vi "log analysis_gps.vi"() -> ()   [LabVIEW 2018] (continued)
log_raw\tgps_raw\t\tsystem status\tnormal 2 28.300000 0 0\trobot status\t14.669720\t18.434430\t9.580100\t-0.442703\t-1.332140\t56.640484\t0.481000\t-0.012000\n\t\n15:06:21.6\tlog_raw\tgps_raw\t\tsystem status\tnormal 2 28.300000 0 0\trobot status\t14.797529\t18.634109\t9.573000\t-0.410192\t-1.362528\t56.475857\t0.491000\t-0.012000\n\t\n15:06:22.1\tlog_raw\tgps_raw\t\tsystem status\tnormal 2 28.300000 0 0\trobot status\t14.927663\t18.831915\t9.567300\t-0.251703\t-1.268455\t56.075924\t0.492000\t-0.025000\n\t\n15:06:22.6\tlog_raw\tgps_raw\t\tsystem status\tnormal 2 28.200000 0 0\trobot status\t15.059315\t19.031378\t9.560500\t-0.198157\t-1.501771\t56.406784\t0.493000\t-0.027000\n\t\n15:06:23.1\tlog_raw\tgps_raw\t\tsystem status\tnormal 2 28.300000 0 0\trobot status\t15.196538\t19.238415\t9.553100\t-0.161311\t-1.683922\t55.984398\t0.499000\t-0.017000\n\t\n15:06:23.6\tlog_raw\tgps_raw\t\tsystem status\tnormal 2 28.300000 0 0\trobot status\t15.328121\t19.432271\t9.546000\t-0.255888\t-1.624208\t55.884857\t0.485000\t-0.045000\n\t\n15:06:24.1\tlog_raw\tgps_raw\t\tsystem status\tnormal 2 28.300000 0 0\trobot status\t15.462626\t19.627022\t9.539100\t-0.210675\t-1.326281\t55.617352\t0.516000\t-0.008000\n\t\n15:06:24.6\tlog_raw\tgps_raw\t\tsystem status\tnormal 2 28.300000 0 0\trobot status\t15.603892\t19.828177\t9.530800\t-0.413985\t-1.434365\t55.397999\t0.465000\t-0.076000\n\t\n15:06:25.1\tlog_raw\tgps_raw\t\tsystem status\tnormal 2 28.200000 0 0\trobot status\t15.741500\t20.019302\t9.525900\t-0.572236\t-1.445230\t54.718037\t0.467000\t-0.089000\n\t\n15:06:25.6\tlog_raw\tgps_raw\t\tsystem status\tnormal 2 28.200000 0 0\trobot status\t15.882218\t20.207334\t9.519900\t-0.498192\t-1.514932\t54.414841\t0.447000\t-0.134000\n\t\n15:06:26.1\tlog_raw\tgps_raw\t\tsystem status\tnormal 2 28.200000 0 0\trobot status\t16.023898\t20.392153\t9.513000\t-0.472443\t-1.210385\t53.436024\t0.532000\t0.043000\n\t\n15:06:26.7\tlog_raw\tgps_raw\t\tsystem status\tnormal 2 28.200000 0 0\trobot status\t16.171592\t20.578219\t9.506200\t-0.708328\t-1.308049\t52.570660\t0.594000\t0.124000\n\t\n15:06:27.1\tlog_raw\tgps_raw\t\tsystem status\tnormal 2 28.200000 0 0\trobot status\t16.321970\t20.758672\t9.499000\t-0.603389\t-1.161147\t50.202438\t0.716000\t0.307000\n\t\n15:06:27.7\tlog_raw\tgps_raw\t\tsystem status\tnormal 2 28.200000 0 0\trobot status\t16.472637\t20.937047\t9.494000\t-0.823952\t-1.192068\t49.516270\t0.549000\t0.052000\n\t\n15:06:28.2\tlog_raw\tgps_raw\t\tsystem status\tnormal 2 28.300000 0 0\trobot status\t16.626209\t21.110847\t9.487200\t-0.618338\t-1.040485\t49.357948\t0.445000\t-0.079000\n\t\n15:06:28.7\tlog_raw\tgps_raw\t\tsystem status\tnormal 2 28.300000 0 0\trobot status\t16.782273\t21.286651\t9.481200\t-0.644616\t-1.219018\t49.316982\t0.467000\t-0.020000\n\t\n15:06:29.2\tlog_raw\tgps_raw\t\tsystem status\tnormal 2 28.300000 0 0\trobot status\t16.937583\t21.455267\t9.475200\t-0.611529\t-1.254126\t50.028496\t0.494000\t0.009000\n\t\n15:06:29.7\tlog_raw\tgps_raw\t\tsystem status\tnormal 2 28.300000 0 0\trobot status\t17.093303\t21.621011\t9.474500\t-0.765682\t-0.913837\t48.514305\t0.492000\t0.019000\n\t\n15:06:30.2\tlog_raw\tgps_raw\t\tsystem status\tnormal 2 28.200000 0 0\trobot status\t17.247377\t21.778171\t9.473400\t-0.418232\t-0.521781\t48.645527\t0.503000\t0.018000\n\t\n15:06:30.7\tlog_raw\tgps_raw\t\tsystem status\tnormal 2 28.300000 0 0\trobot status\t17.414327\t21.954053\t9.468700\t-0.366987\t-0.668392\t48.759113\t0.491000\t0.027000\n\t\n15:06:31.2\tlog_raw\tgps_raw\t\tsystem status\tnormal 2 28.300000 0 0\trobot status\t17.576209\t22.121930\t9.465900\t-0.344665\t-0.985004\t48.117779\t0.514000\t0.007000\n\t\n15:06:31.7\tlog_raw\tgps_raw\t\tsystem status\tnormal 2 28.200000 0 0\trobot status\t17.741651\t22.297663\t9.462100\t-0.296414\t-1.204172\t48.951267\t0.600000\t-0.140000\n\t\n15:06:32.2\tlog_raw\tgps_raw\t\tsystem status\tnormal 2 28.200000 0 0\trobot status\t17.899739\t22.464471\t9.457900\t-0.150727\t-1.166923\t49.356468\t0.469000\t0.059000\n\t\n15:06:32.7\tlog_raw\tgps_raw\t\tsystem status\tnormal 2 28.100000 0 0\trobot status\t18.056766\t22.634728\t9.453400\t-0.116821\t-1.019282\t49.798592\t0.340000\t0.260000\n\t\n15:06:33.2\tlog_raw\tgps_raw\t\tsystem status\tnormal 2 28.100000 0 0\trobot status\t18.210251\t22.807417\t9.449800\t-0.101973\t-1.178444\t51.238773\t0.429000\t0.127000\n\t\n15:06:33.7\tlog_raw\tgps_raw\t\tsystem status\tnormal 2 28.000000 0 0\trobot status\t18.356919\t22.986067\t9.447300\t-0.277614\t-0.965312\t52.540962\t0.440000\t0.150000\n\t\n15:06:34.2\tlog_raw\tgps_raw\t\tsystem status\tnormal 2 28.000000 0 0\trobot status\t18.501103\t23.165006\t9.443600\t-0.171265\t-0.728076\t53.288834\t0.541000\t-0.049000\n\t\n15:06:34.7\tlog_raw\tgps_raw\t\tsystem status\tnormal 2 28.000000 0 0\trobot status\t18.643616\t23.349578\t9.441700\t0.001085\t-0.423099\t53.132992\t0.514000\t0.022000\n\t\n15:06:35.2\tlog_raw\tgps_raw\t#INSPVAXA,USB3,0,46.0,FINESTEERING,2107,281213.200,02000000,471d,15824;INS_ALIGNMENT_COMPLETE,INS_RTKFIXED,37.37034248828,126.72104733937,9.4372,22.3000,0.3538,0.2828,-0.0066,-0.047417832,-0.921096581,33.030780254,0.4120,0.2924,0.5519,0.1133,0.0939,0.0858,0.2818,0.2696,4.9671,0f000001,0*5574abbc\n\tsystem status\tnormal 2 28.000000 0 0\trobot status\t18.799365\t23.561095\t9.437200\t-0.047418\t-0.921097\t53.638321\t0.558000\t-0.089000\n\t\n15:06:35.7\tlog_raw\tgps_raw\t\tsystem status\tnormal 2 28.000000 0 0\trobot status\t18.923249\t23.736439\t9.433200\t-0.135144\t-1.055623\t54.359356\t0.640000\t-0.194000\n\t\n15:06:36.2\tlog_raw\tgps_raw\t\tsystem status\tnormal 2 28.100000 0 0\trobot status\t19.058113\t23.933319\t9.428500\t-0.205469\t-1.114172\t54.854160\t0.442000\t0.079000\n\t\n15:06:36.7\tlog_raw\tgps_raw\t\tsystem status\tnormal 2 28.100000 0 0\trobot status\t19.188419\t24.132723\t9.424800\t-0.121815\t-0.847459\t55.364796\t0.450000\t0.092000\n\t\n15:06:37.2\tlog_raw\tgps_raw\t#INSPVAXA,USB3,0,45.5,FINESTEERING,2107,281215.200,02000000,471d,15824;INS_ALIGNMENT_COMPLETE,INS_RTKFIXED,37.37034967081,126.72105335114,9.4206,22.3000,0.3913,0.2859,-0.0158,-0.209950038,-1.067150096,30.856231444,0.4131,0.2932,0.5613,0.1129,0.0941,0.0863,0.2814,0.2689,4.9698,0f000001,0*15a1dcfe\n\tsystem status\tnormal 2 28.200000 0 0\trobot status\t19.331878\t24.358244\t9.420600\t-0.209950\t-1.067150\t56.490650\t0.418000\t0.124000\n\t\n15:06:37.7\tlog_raw\tgps_raw\t\tsystem status\tnormal 2 28.200000 0 0\trobot status\t19.448752\t24.543859\t9.415800\t-0.435181\t-1.200392\t56.363674\t0.656000\t-0.251000\n\t\n15:06:38.2\tlog_raw\tgps_raw\t\tsystem status\tnormal 2 28.200000 0 0\trobot status\t19.578892\t24.747485\t9.410400\t-0.394118\t-1.104838\t56.147427\t0.483000\t0.009000\n\t\n15:06:38.7\tlog_raw\tgps_raw\t\tsystem status\tnormal 2 28.200000 0 0\trobot status\t19.708910\t24.951700\t9.408000\t-0.473816\t-0.971366\t56.946445\t0.453000\t0.039000\n\t\n15:06:39.2\tlog_raw\tgps_raw\t\tsystem status\tnormal 2 28.200000 0 0\trobot status\t19.839004\t25.154821\t9.405200\t-0.424478\t-1.089783\t55.912186\t0.480000\t0.003000\n\t\n15:06:39.7\tlog_raw\tgps_raw\t#INSPVAXA,USB3,0,47.5,FINESTEERING,2107,281217.700,02000000,471d,15824;INS_ALIGNMENT_COMPLETE,INS_RTKFIXED,37.37035891275,126.72106070272,9.4027,22.3000,0.3907,0.2751,-0.0370,-0.475151732,-0.956253222,31.086527744,0.4118,0.2907,0.5637,0.1115,0.0927,0.0836,0.2812,0.2687,4.9728,0f000001,0*c5b8ff8b\n\tsystem status\tnormal 2 28.300000 0 0\trobot status\t19.983069\t25.383955\t9.402700\t-0.475152\t-0.956253\t55.553867\t0.493000\t-0.013000\n\t\n15:06:40.2\tlog_raw\tgps_raw\t\tsystem status\tnormal 2 28.300000 0 0\trobot status\t20.097932\t25.563951\t9.402700\t-0.538281\t-0.688897\t56.219219\t0.499000\t-0.015000\n\t\n15:06:40.7\tlog_raw\tgps_raw\t#INSPVAXA,USB3,0,41.5,FINESTEERING,2107,281218.700,02000000,471d,15824;INS_ALIGNMENT_COMPLETE,INS_RTKFIXED,37.37036254864,126.72106366487,9.4005,22.3000,0.3951,0.2706,-0.0129,-0.403197852,-0.697835271,31.463679771,0.4109,0.2895,0.5628,0.1119,0.0933,0.0832,0.2811,0.2686,4.9743,0f000001,0*95cb54ca\n\tsystem status\tnormal 2 28.200000 0 0\trobot status\t20.245451\t25.787482\t9.400500\t-0.403198\t-0.697835\t55.319050\t0.493000\t-0.022000\n\t\n15:06:41.2\tlog_raw\tgps_raw\t\tsystem status\tnormal 2 28.200000 0 0\trobot status\t20.362973\t25.969116\t9.399600\t-0.606996\t-0.535913\t56.163181\t0.494000\t-0.027000\n\t\n15:06:41.7\tlog_raw\tgps_raw\t\tsystem status\tnormal 2 28.300000 0 0\trobot status\t20.493689\t26.170169\t9.401200\t-0.861722\t-0.670275\t55.873943\t0.502000\t-0.039000\n\t\n15:06:42.2\tlog_raw\tgps_raw\t\tsystem status\tnormal 2 28.300000 0 0\trobot status\t20.632432\t26.380765\t9.400800\t-0.844302\t-0.845400\t54.259411\t0.490000\t-0.026000\n\t\n15:06:42.7\tlog_raw\tgps_raw\t#INSPVAXA,USB3,0,45.0,FINESTEERING,2107,281220.700,02000000,471d,15824;INS_ALIGNMENT_COMPLETE,INS_RTKFIXED,37.37036990061,126.72106971349,9.4025,22.3000,0.4109,0.2911,0.0071,-0.800702945,-0.878644990,32.737645043,0.4094,0.2870,0.5571,0.1117,0.0929,0.0807,0.2810,0.2681,4.9772,0f000001,0*67c969e8\n\tsystem status\tnormal 2 28.200000 0 0\trobot status\t20.781228\t26.603436\t9.402500\t-0.800703\t-0.878645\t54.810455\t0.511000\t-0.023000\n\t\n15:06:43.2\tlog_raw\tgps_raw\t#INSPVAXA,USB3,0,42.5,FINESTEERING,2107,281221.200,02000000,471d,15824;INS_ALIGNMENT_COMPLETE,INS_RTKFIXED,37.37037172466,126.72107126440,9.4031,22.3000,0.4112,0.2890,-0.0190,-0.732165245,-0.750314239,33.130718379,0.4093,0.2853,0.5533,0.1117,0.0926,0.0797,0.2808,0.2678,4.9785,0f000001,0*69bb78c8\n\tsystem status\tnormal 2 28.200000 0 0\trobot status\t20.918605\t26.805878\t9.403100\t-0.732165\t-0.750314\t53.298634\t0.499000\t-0.017000\n\t\n15:06:43.7\tlog_raw\tgps_raw\t\tsystem status\tnormal 2 28.200000 0 0\trobot status\t21.046031\t26.987368\t9.403400\t-0.631340\t-0.757970\t54.422825\t0.498000\t-0.011000\n\t\n15:06:44.2\tlog_raw\tgps_raw\t\tsystem status\tnormal 2 28.200000 0 0\trobot status\t21.184536\t27.183020\t9.401900\t-0.652815\t-0.900259\t53.609329\t0.446000\t-0.086000\n\t\n15:06:44.7\tlog_raw\tgps_raw\t\tsystem status\tnormal 2 28.300000 0 0\trobot status\t21.325364\t27.376921\t9.402200\t-0.694030\t-0.892817\t53.428085\t0.543000\t0.053000\n\t\n15:06:45.2\tlog_raw\tgps_raw\t\tsystem status\tnormal 2 28.200000 0 0\trobot status\t21.469638\t27.569712\t9.402700\t-0.559469\t-0.735313\t52.854458\t0.654000\t0.219000\n\t\n15:06:45.7\tlog_raw\tgps_raw\t\tsystem status\tnormal 2 28.200000 0 0\trobot status\t21.616373\t27.759644\t9.402600\t-0.651466\t-0.781679\t51.706299\t0.653000\t0.201000\n\t\n15:06:46.2\tlog_raw\tgps_raw\t\tsystem status\tnormal 2 28.200000 0 0\trobot status\t21.764966\t27.945708\t9.403800\t-0.588520\t-0.809740\t51.243496\t0.562000\t0.068000\n\t\n15:06:46.7\tlog_raw\tgps_raw\t#INSPVAXA,USB3,0,47.0,FINESTEERING,2107,281224.700,02000000,471d,15824;INS_ALIGNMENT_COMPLETE,INS_RTKFIXED,37.37038378890,126.72108266803,9.4041,22.3000,0.3641,0.2986,-0.0101,-0.663611718,-0.597748671,37.087466475,0.4089,0.2830,0.5420,0.1122,0.0925,0.0797,0.2801,0.2667,4.9821,0f000001,0*d2353e58\n\tsystem status\tnormal 2 28.200000 0 0\trobot status\t21.928720\t28.144820\t9.404100\t-0.663612\t-0.597749\t50.318630\t0.431000\t-0.109000\n\t\n15:06:47.2\tlog_raw\tgps_raw\t\tsystem status\tnormal 2 28.200000 0 0\trobot status\t22.067987\t28.309838\t9.404300\t-0.492724\t-0.435729\t50.359184\t0.490000\t-0.020000\n\t\n15:06:47.7\tlog_raw\tgps_raw\t#INSPVAXA,USB3,0,49.0,FINESTEERING,2107,281225.700,02008000,471d,15824;INS_ALIGNMENT_COMPLETE,INS_RTKFIXED,37.37038703252,126.72108609198,9.4018,22.3000,0.3794,0.3187,-0.0066,-0.623620259,-0.927536897,37.861250178,0.4087,0.2831,0.5398,0.1124,0.0928,0.0802,0.2799,0.2664,4.9834,0f000001,0*fbb2d3ef\n\tsystem status\tnormal 2 28.200000 0 0\trobot status\t22.232008\t28.504811\t9.401800\t-0.623620\t-0.927537\t49.387749\t0.499000\t-0.009000\n\t\n15:06:48.2\tlog_raw\tgps_raw\t\tsystem status\tnormal 2 28.200000 0 0\trobot status\t22.365284\t28.660268\t9.401600\t-0.754168\t-1.309650\t49.058773\t0.479000\t0.009000\n\t\n15:06:48.7\tlog_raw\tgps_raw\t#INSPVAXA,USB3,0,46.0,FINESTEERING,2107,281226.700,02008000,471d,15824;INS_ALIGNMENT_COMPLETE,INS_RTKFIXED,37.37039019698,126.72108954824,9.4032,22.3000,0.3584,0.3195,-0.0134,-0.717043811,-1.235643045,38.442839555,0.4087,0.2833,0.5380,0.1119,0.0921,0.0796,0.2798,0.2663,4.9847,0f000001,0*b92bfc16\n\tsystem status\tnormal 2 28.300000 0 0\trobot status\t22.538157\t28.856016\t9.403200\t-0.717044\t-1.235643\t49.151516\t0.493000\t0.009000\n\t\n15:06:49.2\tlog_raw\tgps_raw\t\tsystem status\tnormal 2 28.300000 0 0\trobot status\t22.678868\t29.011378\t9.400800\t-0.623594\t-1.018401\t49.199638\t0.496000\t0.016000\n\t\n15:06:49.7\tlog_raw\tgps_raw\t#INSPVAXA,USB3,0,43.5,FINESTEERING,2107,281227.700,02008000,471d,15824;INS_ALIGNMENT_COMPLETE,INS_RTKFIXED,37.37039325687,126.72109307012,9.3982,22.3000,0.3516,0.3055,0.0005,-0.625802804,-1.271897010,38.869801853,0.4083,0.2827,0.5361,0.1122,0.0924,0.0800,0.2797,0.2662,4.9860,0f000001,0*e8201bda\n\tsystem status\tnormal 2 28.300000 0 0\trobot status\t22.850120\t29.195616\t9.398200\t-0.625803\t-1.271897\t48.625996\t0.493000\t0.011000\n\t\n15:06:50.2\tlog_raw\tgps_raw\t#INSPVAXA,USB3,0,44.5,FINESTEERING,2107,281228.200,02008000,471d,15824;INS_ALIGNMENT_COMPLETE,INS_RTKFIXED,37.37039486129,126.72109491850,9.3967,22.3000,0.3668,0.3505,-0.0187,-0.688902140,-1.335982228,38.955777552,0.4076,0.2823,0.5343,0.1119,0.0921,0.0794,0.2796,0.2660,4.9872,0f000001,0*8630753c\n\tsystem status\tnormal 2 28.300000 0 0\trobot status\t23.013846\t29.373682\t9.396700\t-0.688902\t-1.335982\t48.590324\t0.506000\t0.017000\n\t\n15:06:50.7\tlog_raw\tgps_raw\t\tsystem status\tnormal 2 28.200000 0 0\trobot status\t23.159327\t29.527717\t9.396200\t-0.419608\t-1.258090\t48.867809\t0.419000\t0.117000\n\t\n15:06:51.2\tlog_raw\tgps_raw\t#INSPVAXA,USB3,0,42.5,FINESTEERING,2107,281229.200,02008000,471d,15824;INS_ALIGNMENT_COMPLETE,INS_RTKFIXED,37.37039793167,126.72109852773,9.3953,22.3000,0.3279,0.2928,-0.0255,-0.253376052,-0.991820405,38.455195972,0.4075,0.2825,0.5342,0.1118,0.0921,0.0790,0.2795,0.2658,4.9885,0f000001,0*8eb4cf39\n\tsystem status\tnormal 2 28.200000 0 0\trobot status\t23.333546\t29.714446\t9.395300\t-0.253376\t-0.991820\t50.004395\t0.514000\t-0.011000\n\t\n15:06:51.7\tlog_raw\tgps_raw\t#INSPVAXA,USB3,0,42.5,FINESTEERING,2107,281229.700,02008000,471d,15824;INS_ALIGNMENT_COMPLETE,INS_RTKFIXED,37.37039951050,126.72110026434,9.3940,22.3000,0.3314,0.2910,-0.0037,-0.337455745,-0.999192864,37.610056402,0.4075,0.2825,0.5342,0.1118,0.0921,0.0790,0.2795,0.2658,4.9885,0f000001,0*825b5af1\n\tsystem status\tnormal 2 28.100000 0 0\trobot status\t23.487372\t29.889671\t9.394000\t-0.337456\t-0.999193\t51.128315\t0.533000\t-0.026000\n\t\n15:06:52.2\tlog_raw\tgps_raw\t\tsystem status\tnormal 2 28.100000 0 0\trobot status\t23.625713\t30.049641\t9.393400\t-0.271176\t-1.130819\t51.201752\t0.436000\t0.112000\n\t\n15:06:52.7\tlog_raw\tgps_raw\t#INSPVAXA,USB3,0,48.0,FINESTEERING,2107,281230.700,02000000,471d,15824;INS_ALIGNMENT_COMPLETE,INS_RTKFIXED,37.37040272369,126.72110367197,9.3887,22.3000,0.3216,0.2986,0.0135,-0.067201953,-1.333373394,35.463092015,0.4076,0.2834,0.5341,0.1119,0.0922,0.0790,0.2794,0.2655,4.9897,0f000001,0*735b730c\n\tsystem status\tnormal 2 28.000000 0 0\trobot status\t23.789214\t30.246285\t9.388700\t-0.067202\t-1.333373\t52.971828\t0.415000\t0.157000\n\t\n15:06:53.2\tlog_raw\tgps_raw\t#INSPVAXA,USB3,0,47.0,FINESTEERING,2107,281231.200,02000000,471d,15824;INS_ALIGNMENT_COMPLETE,INS_RTKFIXED,37.37040437272,126.72110529054,9.3853,22.3000,0.3713,0.2903,-0.0029,0.017258070,-1.218794572,34.494374429,0.4079,0.2828,0.5329,0.1115,0.0914,0.0786,0.2791,0.2650,4.9910,0f000001,0*8245b70f\n\tsystem status\tnormal 2 28.000000 0 0\trobot status\t23.932585\t30.429301\t9.385300\t0.017258\t-1.218795\t53.613220\t0.408000\t0.170000\n\t\n15:06:53.7\tlog_raw\tgps_raw\t\tsystem status\tnormal 2 28.100000 0 0\trobot status\t24.056260\t30.599212\t9.380600\t-0.026863\t-1.285130\t55.009392\t0.549000\t-0.026000\n\t\n15:06:54.2\tlog_raw\tgps_raw\t#INSPVAXA,USB3,0,48.0,FINESTEERING,2107,281232.200,02000000,471d,15824;INS_ALIGNMENT_COMPLETE,INS_RTKFIXED,37.37040781109,126.72110834724,9.3744,22.3000,0.3888,0.2640,-0.0077,-0.124217348,-1.394698716,32.685462252,0.4076,0.2824,0.5319,0.1108,0.0907,0.0781,0.2788,0.2646,4.9925,0f000001,0*3486c657\n\tsystem status\tnormal 2 28.000000 0 0\trobot status\t24.203342\t30.810907\t9.374400\t-0.124217\t-1.394699\t55.228851\t0.325000\t0.271000\n\t\n15:06:54.7\tlog_raw\tgps_raw\t#INSPVAXA,USB3,0,48.0,FINESTEERING,2107,281232.700,02000000,471d,15824;INS_ALIGNMENT_COMPLETE,INS_RTKFIXED,37.37040957768,126.72110983569,9.3683,22.3000,0.3693,0.2541,-0.0175,-0.035465033,-1.483738306,31.883679858,0.4076,0.2824,0.5319,0.1108,0.0907,0.0781,0.2788,0.2646,4.9925,0f000001,0*4cf861df\n\tsystem status\tnormal 2 28.100000 0 0\trobot status\t24.335187\t31.006971\t9.368300\t-0.035465\t-1.483738\t55.660633\t0.385000\t0.203000\n\t\n15:06:55.2\tlog_raw\tgps_raw\t#INSPVAXA,USB3,0,42.5,FINESTEERING,2107,281233.200,02000000,471d,15824;INS_ALIGNMENT_COMPLETE,INS_RTKFIXED,37.37041136091,126.72111130172,9.3607,22.3000,0.3896,0.2699,-0.0002,0.128694926,-1.559285557,31.391109709,0.4078,0.2816,0.5308,0.1112,0.0913,0.0791,0.2786,0.2642,4.9941,0f000001,0*46ab5c2a\n\tsystem status\tnormal 2 28.100000 0 0\trobot status\t24.465045\t31.204881\t9.360700\t0.128695\t-1.559286\t56.024055\t0.428000\t0.097000\n\t\n15:06:55.7\tlog_raw\tgps_raw\t#INSPVAXA,USB3,0,42.5,FINESTEERING,2107,281233.700,02000000,471d,15824;INS_ALIGNMENT_COMPLETE,INS_RTKFIXED,37.37041314780,126.72111272697,9.3553,22.3000,0.3924,0.2487,-0.0281,0.163758724,-1.359425913,31.096827482,0.4078,0.2816,0.5308,0.1112,0.0913,0.0791,0.2786,0.2642,4.9941,0f000001,0*d64e85f7\n\tsystem status\tnormal 2 28.100000 0 0\trobot status\t24.591291\t31.403198\t9.355300\t0.163759\t-1.359426\t56.679836\t0.391000\t0.162000\n\t\n15:06:56.2\tlog_raw\tgps_raw\t#INSPVAXA,USB3,0,47.0,FINESTEERING,2107,281234.200,02000000,471d,15824;INS_ALIGNMENT_COMPLETE,INS_RTKFIXED,37.37041499218,126.72111417057,9.3481,22.3000,0.4102,0.2507,-0.0208,-0.006261741,-1.350650653,30.806533983,0.4074,0.2813,0.5302,0.1115,0.0918,0.0799,0.2784,0.2639,4.9958,0f000001,0*5fc48718\n\tsystem status\tnormal 2 28.200000 0 0\trobot status\t24.719163\t31.607896\t9.348100\t-0.006262\t-1.350651\t55.675377\t0.414000\t0.126000\n\t\n15:06:56.7\tlog_raw\tgps_raw\t#INSPVAXA,USB3,0,47.0,FINESTEERING,2107,281234.700,02000000,471d,15824;INS_ALIGNMENT_COMPLETE,INS_RTKFIXED,37.37041679366,126.72111558413,9.3430,22.3000,0.3853,0.2462,-0.0143,0.055762675,-1.167743160,30.720625161,0.4074,0.2813,0.5302,0.1115,0.0918,0.0799,0.2784,0.2639,4.9958,0f000001,0*9a377d3f\n\tsystem status\tnormal 2 28.200000 0 0\trobot status\t24.844374\t31.807832\t9.343000\t0.055763\t-1.167743\t57.176826\t0.404000\t0.142000\n\t\n15:06:57.2\tlog_raw\tgps_raw\t#INSPVAXA,USB3,0,48.0,FINESTEERING,2107,281235.200,02000000,471d,15824;INS_ALIGNMENT_COMPLETE,INS_RTKFIXED,37.37041862614,126.72111704485,9.3377,22.3000,0.3985,0.2540,-0.0201,0.294289103,-1.099012992,30.736583565,0.4070,0.2811,0.5299,0.1117,0.0922,0.0805,0.2783,0.2638,4.9972,0f000001,0*a95814ac\n\tsystem status\tnormal 2 28.200000 0 0\trobot status\t24.973762\t32.011208\t9.337700\t0.294289\t-1.099013\t57.295681\t0.594000\t-0.146000\n\t\n15:06:57.7\tlog_raw\tgps_raw\t\tsystem status\tnormal 2 28.300000 0 0\trobot status\t25.089206\t32.194708\t9.334000\t0.121491\t-1.212612\t57.047039\t0.475000\t0.029000\n\t\n15:06:58.2\tlog_raw\tgps_raw\t#INSPVAXA,USB3,0,44.0,FINESTEERING,2107,281236.200,02000000,471d,15824;INS_ALIGNMENT_COMPLETE,INS_RTKFIXED,37.37042228816,126.72111996191,9.3297,22.3000,0.3967,0.2694,0.0011,0.104811084,-1.415486457,30.958501575,0.4068,0.2811,0.5298,0.1121,0.0927,0.0811,0.2782,0.2636,4.9988,0f000001,0*e69fee41\n\tsystem status\tnormal 2 28.200000 0 0\trobot status\t25.232150\t32.417635\t9.329700\t0.104811\t-1.415486\t57.066120\t0.489000\t-0.015000\n\t\n15:06:58.7\tlog_raw\tgps_raw\t#INSPVAXA,USB3,0,44.0,FINESTEERING,2107,281236.700,02000000,471d,15824;INS_ALIGNMENT_COMPLETE,INS_RTKFIXED,37.37042410585,126.72112143606,9.3271,22.3000,0.4148,0.2479,-0.0173,0.069526094,-1.244882003,31.226949687,0.4068,0.2811,0.5298,0.1121,0.0927,0.0811,0.2782,0.2636,4.9988,0f000001,0*974dad1a\n\tsystem status\tnormal 2 28.200000 0 0\trobot status\t25.362728\t32.619371\t9.327100\t0.069526\t-1.244882\t57.115856\t0.494000\t-0.018000\n\t\n15:06:59.2\tlog_raw\tgps_raw\t#INSPVAXA,USB3,0,45.5,FINESTEERING,2107,281237.200,02000000,471d,15824;INS_ALIGNMENT_COMPLETE,INS_RTKFIXED,37.37042595037,126.72112294514,9.3228,22.3000,0.4143,0.2621,-0.0195,0.018984845,-1.146574514,31.412832351,0.4068,0.2809,0.5300,0.1124,0.0929,0.0818,0.2782,0.2635,5.0001,0f000001,0*1b0b7511\n\tsystem status\tnormal 2 28.300000 0 0\trobot status\t25.496400\t32.824083\t9.322800\t0.018985\t-1.146575\t56.291309\t0.494000\t-0.025000\n\t\n15:06:59.7\tlog_raw\tgps_raw\t\tsystem status\tnormal 2 28.300000 0 0\trobot status\t25.616064\t33.008512\t9.318600\t-0.220666\t-1.168167\t55.641972\t0.494000\t-0.031000\n\t\n15:07:00.2\tlog_raw\tgps_raw\t#INSPVAXA,USB3,0,46.0,FINESTEERING,2107,281238.200,02000000,471d,15824;INS_ALIGNMENT_COMPLETE,INS_RTKFIXED,37.37042950556,126.72112589522,9.3162,22.3000,0.4227,0.2698,0.0109,-0.200950173,-1.225682197,31.991269010,0.4072,0.2814,0.5306,0.1126,0.0929,0.0821,0.2781,0.2633,5.0015,0f000001,0*0794d365\n\tsystem status\tnormal 2 28.200000 0 0\trobot status\t25.757713\t33.218654\t9.316200\t-0.200950\t-1.225682\t55.934803\t0.493000\t-0.033000\n\t\n15:07:00.7\tlog_raw\tgps_raw\t#INSPVAXA,USB3,0,46.0,FINESTEERING,2107,281238.700,02000000,471d,15824;INS_ALIGNMENT_COMPLETE,INS_RTKFIXED,37.37043136222,126.72112745012,9.3124,22.3000,0.3943,0.2610,-0.0034,-0.386075100,-1.055396973,32.303525418,0.4072,0.2814,0.5306,0.1126,0.0929,0.0821,0.2781,0.2633,5.0015,0f000001,0*b83f878f\n\tsystem status\tnormal 2 28.300000 0 0\trobot status\t25.895444\t33.424714\t9.312400\t-0.386075\t-1.055397\t55.359413\t0.488000\t-0.027000\n\t\n15:07:01.2\tlog_raw\tgps_raw\t#INSPVAXA,USB3,0,48.0,FINESTEERING,2107,281239.200,02000000,471d,15824;INS_ALIGNMENT_COMPLETE,INS_RTKFIXED,37.37043317421,126.72112899719,9.3082,22.3000,0.4229,0.2915,-0.0051,-0.601506293,-1.130264131,32.679510223,0.4077,0.2817,0.5313,0.1126,0.0927,0.0822,0.2780,0.2630,5.0030,0f000001,0*20b6ea60\n\tsystem status\tnormal 2 28.200000 0 0\trobot status\t26.032481\t33.625817\t9.308200\t-0.601506\t-1.130264\t54.440792\t0.518000\t0.007000\n\t\n15:07:01.7\tlog_raw\tgps_raw\t#INSPVAXA,USB3,0,48.0,FINESTEERING,2107,281239.700,02000000,471d,15824;INS_ALIGNMENT_COMPLETE,INS_RTKFIXED,37.37043494669,126.72113055654,9.3053,22.3000,0.3888,0.2751,0.0114,-0.527038366,-1.080230445,33.250438434,0.4077,0.2817,0.5313,0.1126,0.0927,0.0822,0.2780,0.2630,5.0030,0f000001,0*94791092\n\tsystem status\tnormal 2 28.200000 0 0\trobot status\t26.170605\t33.822534\t9.305300\t-0.527038\t-1.080230\t54.062698\t0.518000\t0.028000\n\t\n15:07:02.2\tlog_raw\tgps_raw\t\tsystem status\tnormal 2 28.200000 0 0\trobot status\t26.298661\t34.004737\t9.302000\t-0.864108\t-1.393350\t52.140862\t0.498000\t-0.021000\n\t\n15:07:02.7\tlog_raw\tgps_raw\t#INSPVAXA,USB3,0,48.5,FINESTEERING,2107,281240.700,02000000,471d,15824;INS_ALIGNMENT_COMPLETE,INS_RTKFIXED,37.37043850253,126.72113379936,9.2976,22.3000,0.4169,0.2904,-0.0141,-0.976451257,-1.265439049,34.098588845,0.4076,0.2813,0.5318,0.1117,0.0919,0.0814,0.2779,0.2627,5.0045,0f000001,0*ee6793dd\n\tsystem status\tnormal 2 28.200000 0 0\trobot status\t26.457849\t34.217177\t9.297600\t-0.976451\t-1.265439\t51.962944\t0.502000\t-0.020000\n\t\n15:07:03.2\tlog_raw\tgps_raw\t#INSPVAXA,USB3,0,46.5,FINESTEERING,2107,281241.200,02000000,471d,15824;INS_ALIGNMENT_COMPLETE,INS_RTKFIXED,37.37044019660,126.72113544542,9.2926,22.3000,0.4279,0.3108,-0.0036,-0.766553513,-1.370370056,34.585070346,0.4075,0.2803,0.5320,0.1109,0.0908,0.0805,0.2778,0.2623,5.0052,0f000001,0*260ccca0\n\tsystem status\tnormal 2 28.200000 0 0\trobot status\t26.603654\t34.405192\t9.292600\t-0.766554\t-1.370370\t52.489170\t0.512000\t-0.019000\n\t\n15:07:03.7\tlog_raw\tgps_raw\t#INSPVAXA,USB3,0,46.5,FINESTEERING,2107,281241.700,02000000,471d,15824;INS_ALIGNMENT_COMPLETE,INS_RTKFIXED,37.37044183342,126.72113705465,9.2914,22.3000,0.3729,0.2861,0.0243,-0.736192584,-1.169550873,35.066959350,0.4075,0.2803,0.5320,0.1109,0.0908,0.0805,0.2778,0.2623,5.0052,0f000001,0*7de3fdbf\n\tsystem status\tnormal 2 28.200000 0 0\trobot status\t26.746197\t34.586853\t9.291400\t-0.736193\t-1.169551\t52.282486\t0.488000\t-0.006000\n\t\n15:07:04.2\tlog_raw\tgps_raw\t#INSPVAXA,USB3,0,46.5,FINESTEERING,2107,281242.200,02000000,471d,15824;INS_ALIGNMENT_COMPLETE,INS_RTKFIXED,37.37044357732,126.72113877934,9.2913,22.3000,0.3995,0.2989,-0.0112,-0.773150570,-1.240971766,35.457586747,0.4072,0.2799,0.5319,0.1103,0.0904,0.0797,0.2776,0.2620,5.0062,0f000001,0*047104d0\n\tsystem status\tnormal 2 28.300000 0 0\trobot status\t26.898968\t34.780399\t9.291300\t-0.773151\t-1.240972\t51.430470\t0.510000\t0.004000\n\t\n15:07:04.7\tlog_raw\tgps_raw\t#INSPVAXA,USB3,0,46.5,FINESTEERING,2107,281242.700,02000000,471d,15824;INS_ALIGNMENT_COMPLETE,INS_RTKFIXED,37.37044518884,126.72114042326,9.2923,22.3000,0.3596,0.3049,0.0120,-0.827179513,-0.912103368,35.739029632,0.4072,0.2799,0.5319,0.1103,0.0904,0.0797,0.2776,0.2620,5.0062,0f000001,0*089314b8\n\tsystem status\tnormal 2 28.200000 0 0\trobot status\t27.044583\t34.959252\t9.292300\t-0.827180\t-0.912103\t51.825771\t0.473000\t-0.019000\n\t\n15:07:05.2\tlog_raw\tgps_raw\t#INSPVAXA,USB3,0,47.5,FINESTEERING,2107,281243.200,02000000,471d,15824;INS_ALIGNMENT_COMPLETE,INS_RTKFIXED,37.37044682347,126.72114212345,9.2944,22.3000,0.3805,0.3012,0.0098,-0.728489494,-1.051472192,36.148202459,0.4069,0.2798,0.5321,0.1112,0.0916,0.0809,0.2775,0.2618,5.0071,0f000001,0*ab715168\n\tsystem status\tnormal 2 28.300000 0 0\trobot status\t27.195183\t35.140671\t9.294400\t-0.728489\t-1.051472\t51.155540\t0.485000\t-0.022000\n\t\n15:07:05.7\tlog_raw\tgps_raw\t#INSPVAXA,USB3,0,47.5,FINESTEERING,2107,281243.700,02000000,471d,15824;INS_ALIGNMENT_COMPLETE,INS_RTKFIXED,37.37044842257,126.72114379217,9.2929,22.3000,0.3497,0.2949,0.0009,-0.706502684,-0.959221575,36.485073335,0.4069,0.2798,0.5321,0.1112,0.0916,0.0809,0.2775,0.2618,5.0071,0f000001,0*0606f155\n\tsystem status\tnormal 2 28.300000 0 0\trobot status\t27.342996\t35.318146\t9.292900\t-0.706503\t-0.959222\t51.616810\t0.484000\t-0.014000\n\t\n15:07:06.2\tlog_raw\tgps_raw\t#INSPVAXA,USB3,0,48.0,FINESTEERING,2107,281244.200,02000000,471d,15824;INS_ALIGNMENT_COMPLETE,INS_RTKFIXED,37.37045000855,126.72114549963,9.2935,22.3000,0.3813,0.3173,-0.0073,-0.659947391,-1.102241434,36.768615727,0.4069,0.2807,0.5325,0.1118,0.0924,0.0817,0.2773,0.2617,5.0086,0f000001,0*dffaeeda\n\tsystem status\tnormal 2 28.200000 0 0\trobot status\t27.494240\t35.494165\t9.293500\t-0.659947\t-1.102241\t51.626923\t0.495000\t0.002000\n\t\n15:07:06.7\tlog_raw\tgps_raw\t#INSPVAXA,USB3,0,48.0,FINESTEERING,2107,281244.700,02000000,471d,15824;INS_ALIGNMENT_COMPLETE,INS_RTKFIXED,37.37045160181,126.72114725109,9.2936,22.3000,0.3610,0.3198,-0.0165,-0.651308584,-1.162087576,36.974039680,0.4069,0.2807,0.5325,0.1118,0.0924,0.0817,0.2773,0.2617,5.0086,0f000001,0*f70d22ce\n\tsystem status\tnormal 2 28.200000 0 0\trobot status\t27.649381\t35.670991\t9.293600\t-0.651309\t-1.162088\t50.002937\t0.493000\t0.005000\n\t\n15:07:07.2\tlog_raw\tgps_raw\t#INSPVAXA,USB3,0,45.5,FINESTEERING,2107,281245.200,02000000,471d,15824;INS_ALIGNMENT_COMPLETE,INS_RTKFIXED,37.37045318824,126.72114900963,9.2932,22.3000,0.3383,0.3092,0.0249,-0.721431516,-1.066505457,37.188586073,0.4071,0.2814,0.5325,0.1122,0.0928,0.0822,0.2772,0.2616,5.0103,0f000001,0*ccafe7f7\n\tsystem status\tnormal 2 28.200000 0 0\trobot status\t27.805150\t35.847060\t9.293200\t-0.721432\t-1.066505\t49.771038\t0.493000\t0.009000\n\t\n15:07:07.7\tlog_raw\tgps_raw\t#INSPVAXA,USB3,0,45.5,FINESTEERING,2107,281245.700,02000000,471d,15824;INS_ALIGNMENT_COMPLETE,INS_RTKFIXED,37.37045471115,126.72115068638,9.2913,22.3000,0.3729,0.3102,-0.0028,-0.841928711,-1.027529391,37.390122228,0.4071,0.2814,0.5325,0.1122,0.0928,0.0822,0.2772,0.2616,5.0103,0f000001,0*6bbac107\n\tsystem status\tnormal 2 28.200000 0 0\trobot status\t27.953674\t36.016079\t9.291300\t-0.841929\t-1.027529\t50.072105\t0.493000\t0.013000\n\t\n15:07:08.2\tlog_raw\tgps_raw\t#INSPVAXA,USB3,0,45.5,FINESTEERING,2107,281246.200,02000000,471d,15824;INS_ALIGNMENT_COMPLETE,INS_RTKFIXED,37.37045637770,126.72115252290,9.2880,22.3000,0.3686,0.3330,-0.0134,-0.785462216,-0.911426514,37.597924060,0.4074,0.2823,0.5331,0.1123,0.0929,0.0823,0.2772,0.2616,5.0118,0f000001,0*adb8b62a\n\tsystem status\tnormal 2 28.300000 0 0\trobot status\t28.116350\t36.201040\t9.288000\t-0.785462\t-0.911427\t49.777924\t0.502000\t0.006000\n\t\n15:07:08.7\tlog_raw\tgps_raw\t#INSPVAXA,USB3,0,45.5,FINESTEERING,2107,281246.700,02000000,471d,15824;INS_ALIGNMENT_COMPLETE,INS_RTKFIXED,37.37045798543,126.72115430749,9.2870,22.3000,0.3687,0.3323,0.0184,-0.822794799,-1.314908192,37.714000338,0.4074,0.2823,0.5331,0.1123,0.0929,0.0823,0.2772,0.2616,5.0118,0f000001,0*e142e69f\n\tsystem status\tnormal 2 28.200000 0 0\trobot status\t28.274426\t36.379473\t9.287000\t-0.822795\t-1.314908\t49.581783\t0.429000\t0.114000\n\t\n15:07:09.2\tlog_raw\tgps_raw\t#INSPVAXA,USB3,0,47.0,FINESTEERING,2107,281247.200,02000000,471d,15824;INS_ALIGNMENT_COMPLETE,INS_RTKFIXED,37.37045959180,126.72115606878,9.2846,22.3000,0.3414,0.3044,0.0046,-0.926007496,-1.283685718,37.475312955,0.4073,0.2824,0.5333,0.1125,0.0929,0.0824,0.2771,0.2615,5.0133,0f000001,0*cd9ecdd0\n\tsystem status\tnormal 2 28.200000 0 0\trobot status\t28.430438\t36.557755\t9.284600\t-0.926007\t-1.283686\t49.614594\t0.411000\t0.126000\n\t\n15:07:09.7\tlog_raw\tgps_raw\t#INSPVAXA,USB3,0,47.0,FINESTEERING,2107,281247.700,02000000,471d,15824;INS_ALIGNMENT_COMPLETE,INS_RTKFIXED,37.37046119890,126.72115783063,9.2839,22.3000,0.3362,0.3158,0.0008,-0.640262260,-1.260973673,36.963677564,0.4073,0.2824,0.5333,0.1125,0.0929,0.0824,0.2771,0.2615,5.0133,0f000001,0*29beb2b2\n\tsystem status\tnormal 2 28.200000 0 0\trobot status\t28.586500\t36.736117\t9.283900\t-0.640262\t-1.260974\t49.771523\t0.633000\t-0.196000\n\t\n15:07:10.2\tlog_raw\tgps_raw\t#INSPVAXA,USB3,0,44.5,FINESTEERING,2107,281248.200,02000000,471d,15824;INS_ALIGNMENT_COMPLETE,INS_RTKFIXED,37.37046280365,126.72115953545,9.2819,22.3000,0.3356,0.2942,0.0022,-0.584668028,-1.162399511,36.175550915,0.4076,0.2828,0.5341,0.1126,0.0930,0.0826,0.2771,0.2613,5.0149,0f000001,0*7d42a3a6\n\tsystem status\tnormal 2 28.100000 0 0\trobot status\t28.737510\t36.914219\t9.281900\t-0.584668\t-1.162400\t50.882935\t0.359000\t0.224000\n\t\n15:07:10.7\tlog_raw\tgps_raw\t#INSPVAXA,USB3,0,44.5,FINESTEERING,2107,281248.700,02000000,471d,15824;INS_ALIGNMENT_COMPLETE,INS_RTKFIXED,37.37046444744,126.72116118616,9.2798,22.3000,0.3405,0.3106,0.0054,-0.632258383,-1.342162283,35.326473382,0.4076,0.2828,0.5341,0.1126,0.0930,0.0826,0.2771,0.2613,5.0149,0f000001,0*74672090\n\tsystem status\tnormal 2 28.000000 0 0\trobot status\t28.883727\t37.096654\t9.279800\t-0.632258\t-1.342162\t51.799076\t0.535000\t-0.028000\n\t\n15:07:11.2\tlog_raw\tgps_raw\t#INSPVAXA,USB3,0,47.0,FINESTEERING,2107,281249.200,02000000,471d,15824;INS_ALIGNMENT_COMPLETE,INS_RTKFIXED,37.37046613756,126.72116281120,9.2778,22.3000,0.3636,0.2914,-0.0245,-0.793213759,-1.308005739,34.279375865,0.4077,0.2829,0.5343,0.1125,0.0927,0.0827,0.2770,0.2611,5.0165,0f000001,0*423f42ab\n\tsystem status\tnormal 2 28.000000 0 0\trobot status\t29.027670\t37.284231\t9.277800\t-0.793214\t-1.308006\t52.646317\t0.372000\t0.211000\n\t\n15:07:11.7\tlog_raw\tgps_raw\t#INSPVAXA,USB3,0,47.0,FINESTEERING,2107,281249.700,02000000,471d,15824;INS_ALIGNMENT_COMPLETE,INS_RTKFIXED,37.37046782429,126.72116439837,9.2744,22.3000,0.3684,0.2690,0.0171,-0.693439264,-1.326725585,33.382125855,0.4077,0.2829,0.5343,0.1125,0.0927,0.0827,0.2770,0.2611,5.0165,0f000001,0*88d26f4b\n\tsystem status\tnormal 2 28.000000 0 0\trobot status\t29.168259\t37.471432\t9.274400\t-0.693439\t-1.326726\t53.713005\t0.381000\t0.191000\n\t\n15:07:12.2\tlog_raw\tgps_raw\t#INSPVAXA,USB3,0,48.5,FINESTEERING,2107,281250.200,02000000,471d,15824;INS_ALIGNMENT_COMPLETE,INS_RTKFIXED,37.37046951993,126.72116592037,9.2722,22.3000,0.3585,0.2583,-0.0083,-0.676233925,-1.068835400,32.415403285,0.4082,0.2827,0.5347,0.1117,0.0917,0.0817,0.2769,0.2609,5.0181,0f000001,0*23e1d120\n\tsystem status\tnormal 2 28.000000 0 0\trobot status\t29.303076\t37.659621\t9.272200\t-0.676234\t-1.068835\t54.528244\t0.438000\t0.126000\n\t\n15:07:12.7\tlog_raw\tgps_raw\t#INSPVAXA,USB3,0,48.5,FINESTEERING,2107,281250.700,02000000,471d,15824;INS_ALIGNMENT_COMPLETE,INS_RTKFIXED,37.37047125659,126.72116740651,9.2700,22.3000,0.3759,0.2852,-0.0005,-0.704418512,-1.024345278,31.769899431,0.4082,0.2827,0.5347,0.1117,0.0917,0.0817,0.2769,0.2609,5.0181,0f000001,0*220f1c57\n\tsystem status\tnormal 2 28.100000 0 0\trobot status\t29.434715\t37.852363\t9.270000\t-0.704419\t-1.024345\t55.178829\t0.360000\t0.206000\n\t\n15:07:13.2\tlog_raw\tgps_raw\t#INSPVAXA,USB3,0,46.0,FINESTEERING,2107,281251.200,02000000,471d,15824;INS_ALIGNMENT_COMPLETE,INS_RTKFIXED,37.37047303421,126.72116889318,9.2673,22.3000,0.3786,0.2715,-0.0144,-0.713801343,-0.929392253,31.230715731,0.4077,0.2824,0.5344,0.1113,0.0913,0.0813,0.2767,0.2607,5.0197,0f000001,0*81e3f7b1\n\tsystem status\tnormal 2 28.100000 0 0\trobot status\t29.566402\t38.049651\t9.267300\t-0.713801\t-0.929392\t55.656151\t0.397000\t0.155000\n\t\n15:07:13.7\tlog_raw\tgps_raw\t#INSPVAXA,USB3,0,46.0,FINESTEERING,2107,281251.700,02000000,471d,15824;INS_ALIGNMENT_COMPLETE,INS_RTKFIXED,37.37047481505,126.72117034620,9.2660,22.3000,0.4016,0.2734,-0.0090,-0.658846991,-1.106608605,30.760952278,0.4077,0.2824,0.5344,0.1113,0.0913,0.0813,0.2767,0.2607,5.0197,0f000001,0*148382ef\n\tsystem status\tnormal 2 28.200000 0 0\trobot status\t29.695108\t38.247296\t9.266000\t-0.658847\t-1.106609\t56.577026\t0.416000\t0.151000\n\t\n15:07:14.2\tlog_raw\tgps_raw\t#DUALANTENNAHEADINGA,USB3,0,47.5,FINESTEERING,2107,281252.200,02000000,d426,15824;SOL_COMPUTED,NARROW_INT,-1.000000000,33.188526154,-13.188842773,0.0,2.061341047,2.951399803,\"631T\",23,11,11,8,04,00,30,03*cb8882ef\n\tsystem status\tnormal 2 28.200000 0 0\trobot status\t29.825447\t38.449907\t9.263000\t-0.634011\t-1.092157\t56.811474\t0.671000\t-0.274000\n\t\n15:07:14.7\tlog_raw\tgps_raw\t#INSPVAXA,USB3,0,47.5,FINESTEERING,2107,281252.700,02000000,471d,15824;INS_ALIGNMENT_COMPLETE,INS_RTKFIXED,37.37047843924,126.72117325955,9.2610,22.3000,0.3921,0.2613,-0.0047,-0.684255773,-1.075453896,30.582940759,0.4074,0.2818,0.5338,0.1112,0.0914,0.0811,0.2766,0.2605,5.0213,0f000001,0*2a48569e\n\tsystem status\tnormal 2 28.200000 0 0\trobot status\t29.953168\t38.649525\t9.261000\t-0.684256\t-1.075454\t57.357277\t0.438000\t0.079000\n\t\n15:07:15.2\tlog_raw\tgps_raw\t#INSPVAXA,USB3,0,43.0,FINESTEERING,2107,281253.200,02000000,471d,15824;INS_ALIGNMENT_COMPLETE,INS_RTKFIXED,37.37048028352,126.72117473138,9.2588,22.3000,0.4035,0.2637,-0.0100,-0.810109039,-1.254597074,30.636904174,0.4069,0.2810,0.5332,0.1116,0.0919,0.0813,0.2766,0.2604,5.0230,0f000001,0*5ad017a3\n\tsystem status\tnormal 2 28.200000 0 0\trobot status\t30.083540\t38.854211\t9.258800\t-0.810109\t-1.254597\t56.410751\t0.552000\t-0.115000\n\t\n15:07:15.7\tlog_raw\tgps_raw\t#INSPVAXA,USB3,0,43.0,FINESTEERING,2107,281253.700,02000000,471d,15824;INS_ALIGNMENT_COMPLETE,INS_RTKFIXED,37.37048209975,126.72117619764,9.2563,22.3000,0.3713,0.2637,0.0057,-0.851136765,-1.427746599,30.748659143,0.4069,0.2810,0.5332,0.1116,0.0919,0.0813,0.2766,0.2604,5.0230,0f000001,0*3581eb98\n\tsystem status\tnormal 2 28.300000 0 0\trobot status\t30.213419\t39.055784\t9.256300\t-0.851137\t-1.427747\t56.524715\t0.475000\t0.005000\n\t\n15:07:16.2\tlog_raw\tgps_raw\t#INSPVAXA,USB3,0,41.5,FINESTEERING,2107,281254.200,02000000,471d,15824;INS_ALIGNMENT_COMPLETE,INS_RTKFIXED,37.37048389322,126.72117766049,9.2543,22.3000,0.4011,0.2685,-0.0017,-0.904192173,-1.398090908,30.961508821,0.4078,0.2816,0.5344,0.1121,0.0926,0.0815,0.2766,0.2603,5.0245,0f000001,0*1f3e2204\n\tsystem status\tnormal 2 28.200000 0 0\trobot status\t30.342996\t39.254831\t9.254300\t-0.904192\t-1.398091\t55.806561\t0.490000\t-0.022000\n\t\n15:07:16.7\tlog_raw\tgps_raw\t#INSPVAXA,USB3,0,41.5,FINESTEERING,2107,281254.700,02000000,471d,15824;INS_ALIGNMENT_COMPLETE,INS_RTKFIXED,37.37048568888,126.72117913940,9.2511,22.3000,0.3906,0.2712,-0.0003,-0.736378348,-1.044906889,31.224322572,0.4078,0.2816,0.5344,0.1121,0.0926,0.0815,0.2766,0.2603,5.0245,0f000001,0*c5f145ca\n\tsystem status\tnormal 2 28.200000 0 0\trobot status\t30.473996\t39.454121\t9.251100\t-0.736378\t-1.044907\t55.483681\t0.495000\t-0.018000\n\t\n15:07:17.2\tlog_raw\tgps_raw\t#INSPVAXA,USB3,0,44.0,FINESTEERING,2107,281255.200,02000000,471d,15824;INS_ALIGNMENT_COMPLETE,INS_RTKFIXED,37.37048748822,126.72118062065,9.2468,22.3000,0.4035,0.2848,0.0108,-0.751779766,-1.053207928,31.437162852,0.4105,0.2861,0.5416,0.1127,0.0935,0.0821,0.2766,0.2602,5.0258,0f000001,0*b06b1cec\n\tsystem status\tnormal 2 28.200000 0 0\trobot status\t30.605202\t39.653820\t9.246800\t-0.751780\t-1.053208\t55.689064\t0.493000\t-0.024000\n\t\n15:07:17.7\tlog_raw\tgps_raw\t#INSPVAXA,USB3,0,44.0,FINESTEERING,2107,281255.700,02000000,471d,15824;INS_ALIGNMENT_COMPLETE,INS_RTKFIXED,37.37048934103,126.72118213039,9.2433,22.3000,0.4087,0.2855,0.0141,-0.905392438,-1.018943356,31.720261979,0.4105,0.2861,0.5416,0.1127,0.0935,0.0821,0.2766,0.2602,5.0258,0f000001,0*e5e8b97b\n\tsystem status\tnormal 2 28.300000 0 0\trobot status\t30.738933\t39.859453\t9.243300\t-0.905392\t-1.018943\t54.921925\t0.493000\t-0.023000\n\t\n15:07:18.2\tlog_raw\tgps_raw\t#INSPVAXA,USB3,0,48.5,FINESTEERING,2107,281256.200,02000000,471d,15824;INS_ALIGNMENT_COMPLETE,INS_RTKFIXED,37.37049116166,126.72118365474,9.2406,22.3000,0.4005,0.2755,-0.0046,-0.741933390,-0.975317507,31.970856097,0.4116,0.2891,0.5469,0.1124,0.0932,0.0816,0.2765,0.2599,5.0273,0f000001,0*39271fda\n\tsystem status\tnormal 2 28.300000 0 0\trobot status\t30.873957\t40.061514\t9.240600\t-0.741933\t-0.975318\t54.901100\t0.495000\t-0.026000\n\t\n15:07:18.7\tlog_raw\tgps_raw\t#INSPVAXA,USB3,0,48.5,FINESTEERING,2107,281256.700,02000000,471d,15824;INS_ALIGNMENT_COMPLETE,INS_RTKFIXED,37.37049294777,126.72118517063,9.2381,22.3000,0.3986,0.2835,-0.0013,-0.674369824,-1.134847367,32.198409844,0.4116,0.2891,0.5469,0.1124,0.0932,0.0816,0.2765,0.2599,5.0273,0f000001,0*38bc1ccb\n\tsystem status\tnormal 2 28.300000 0 0\trobot status\t31.008232\t40.259744\t9.238100\t-0.674370\t-1.134847\t54.718086\t0.491000\t-0.016000\n\t\n15:07:19.2\tlog_raw\tgps_raw\t#INSPVAXA,USB3,0,42.5,FINESTEERING,2107,281257.200,02000000,471d,15824;INS_ALIGNMENT_COMPLETE,INS_RTKFIXED,37.37049476461,126.72118674012,9.2353,22.3000,0.4039,0.2899,0.0228,-0.674986322,-0.804758073,32.620444545,0.4119,0.2902,0.5497,0.1119,0.0926,0.0809,0.2764,0.2596,5.0289,0f000001,0*72dede25\n\tsystem status\tnormal 2 28.200000 0 0\trobot status\t31.147255\t40.461385\t9.235300\t-0.674986\t-0.804758\t54.434986\t0.495000\t-0.006000\n\t\n15:07:19.7\tlog_raw\tgps_raw\t#DUALANTENNAHEADINGA,USB3,0,42.5,FINESTEERING,2107,281257.700,02000000,d426,15824;SOL_COMPUTED,NARROW_INT,-1.000000000,35.851467133,-13.614562988,0.0,0.761796772,1.619968295,\"631T\",20,13,13,10,04,00,30,33*8335f7c7\n\tsystem status\tnormal 2 28.200000 0 0\trobot status\t31.285928\t40.657505\t9.234200\t-0.685458\t-0.867865\t54.148533\t0.518000\t-0.011000\n\t\n15:07:20.2\tlog_raw\tgps_raw\t#DUALANTENNAHEADINGA,USB3,0,50.0,FINESTEERING,2107,281258.200,02000000,d426,15824;SOL_COMPUTED,NARROW_INT,-1.000000000,36.208633423,-13.477111816,0.0,0.769826293,1.626826406,\"631T\",21,13,13,10,04,00,30,33*663662cf\n\tsystem status\tnormal 2 28.300000 0 0\trobot status\t31.427295\t40.854438\t9.231500\t-0.641666\t-0.911342\t53.791367\t0.468000\t-0.060000\n\t\n15:07:20.7\tlog_raw\tgps_raw\t#DUALANTENNAHEADINGA,USB3,0,50.0,FINESTEERING,2107,281258.700,02000000,d426,15824;SOL_COMPUTED,NARROW_INT,-1.000000000,37.583648682,
